vi "dataOrganize_Conversion.vi"(11 "transposed array":dbl[][](array[numeric])) -> (3 "appended array":dbl[][](array[numeric]))   [LabVIEW 2026]
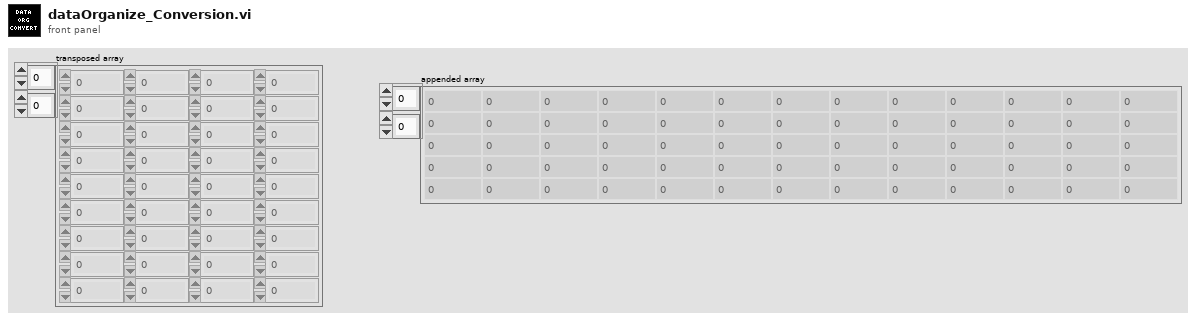
[diagram p1: front panel]
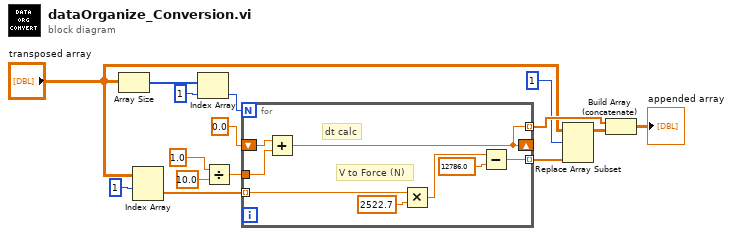
[diagram p0: block diagram]
diagram:
  n1 = Array Size(array="transposed array") -> (size(s)=w1:i32[])
  n2 = Index Array(array="transposed array", index (row)=1) -> (element=w6:dbl[])  [unwired: 1 in]
  n3 = Index Array(array=w1, index=1) -> (element=w14:i32)
  n4 = Divide(x=1.0, y=10.0) -> (x/y=w11:dbl)
  n5 = for {
    N: w14 -> [_]
    shift-right: [w21] -> _
    shift-left: 0.0 -> [w23]
    tunnel: w11 -> [w22]
    tunnel: [w21] -> w9 mode=indexing
    tunnel: w6 -> [w17] mode=indexing
    tunnel: [w16] -> w4 mode=indexing
    # "dt calc"
    # "V to Force (N)"
    n6 = Add(x=w23, y=w22) -> (x+y=w21:dbl)
    n7 = Multiply(x=w17, y=2522.7) -> (x*y=w19:dbl)
    n8 = Subtract(x=w19, y=12786.0) -> (x-y=w16:dbl)
  }
  n9 = Replace Array Subset(array="transposed array", new element=w4, index (row)=1) -> (w3:dbl[][])  [unwired: 1 in]
  n10 = Build Array (concatenate)(w9, w3) -> (→"appended array":dbl[][])
